vi "CanAddKung.vi"(10 "Ponged":u16[](array[numeric]), 11 "Hand":u16[](array[numeric])) -> (1 "TIle":u16, 2 "HandIndex":i16)   [LabVIEW 2025]
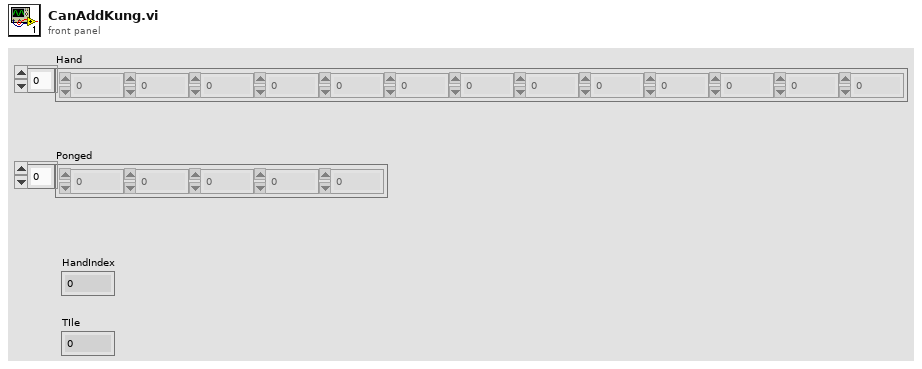
[diagram p1: front panel]
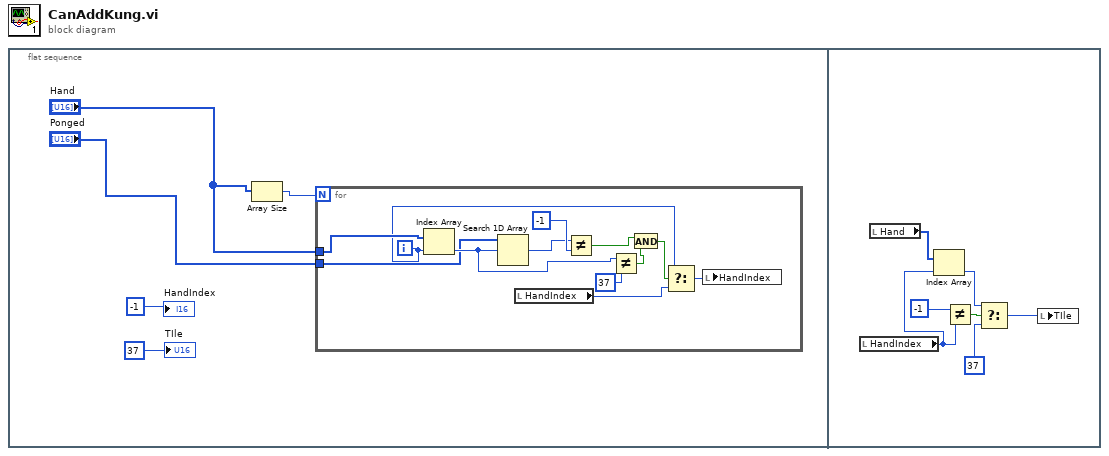
[diagram p0: block diagram]
diagram:
  n1 = flat-sequence {
    frame #0 {
      n2 = Array Size(array="Hand") -> (size(s)=w4:i32)
      n3 = for {
        N: w4 -> [_]
        tunnel: "Ponged" -> [w7]
        tunnel: "Hand" -> [w8]
        i -> [w6]
        n4 = Index Array(array=w8, index=w6) -> (element=w9:u16)
        n5 = Search 1D Array(1D array=w7, element=w9) -> (index of element=w16:i32)  [unwired: 1 in]
        n6 = local read "HandIndex"() -> (w14:i16)
        n7 = Not Equal?(x=w16, y=-1) -> (x != y?=w12:bool)
        n8 = Not Equal?(x=w9, y=37) -> (x != y?=w11:bool)
        n9 = And(x=w12, y=w11) -> (x .and. y?=w13:bool)
        n10 = Select(t=w6, s=w13, f=w14) -> (s? t:f=w15:i32)
        n11 = local write "HandIndex"(w15) -> ()
      }
      "HandIndex" <- -1
      "TIle" <- 37
    }
    frame #1 {
      n12 = local read "HandIndex"() -> (w21:i16)
      n13 = local read "Hand"() -> (w20:u16[])
      n14 = Index Array(array=w20, index=w21) -> (element=w22:u16)
      n15 = Not Equal?(x=-1, y=w21) -> (x != y?=w24:bool)
      n16 = Select(t=w22, s=w24, f=37) -> (s? t:f=w19:i32)
      n17 = local write "TIle"(w19) -> ()
    }
  }
